vi "Write Arbs.vi"(8 "error in (no error)":errorcluster, 10 "Arbs":T1[](array[typedef]), 11 "ArbitraryFunction in":refnum<class "ArbitraryFunction.lvclass">) -> (0 "error out":errorcluster, 3 "ArbitraryFunction out":refnum<class "ArbitraryFunction.lvclass">)   [LabVIEW 2014, in "Functions.lvlib" / "ArbitraryFunction.lvclass"]
uses:
  ArbitraryFunction.lvclass
  TypeDefs/Arbitrary.ctl
  ArbitraryFunction.lvclass/ArbitraryFunction.ctl
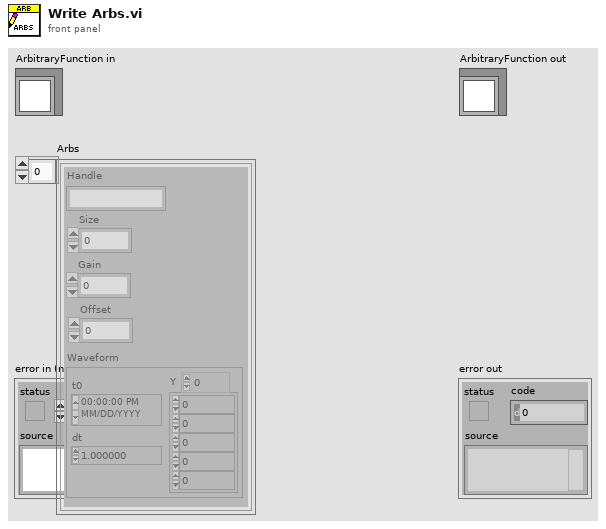
[diagram p1: front panel]
types:
  T1 = typedef "Functions.lvlib/ArbitraryFunction.lvclass/Arbitrary.ctl" = cluster{"Handle":string, "Size":i32, "Gain":dbl, "Offset":dbl, "Waveform":waveform(dbl)}
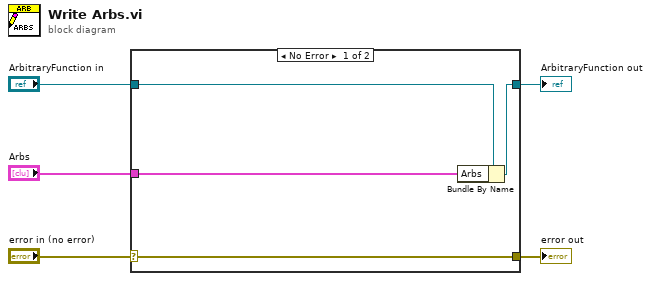
[diagram p0: block diagram]
diagram:
  n1 = case shown="No Error" "error in (no error)" {
    selector: "error in (no error)" -> [w9 w10]
    tunnel: [w9 w10] -> w4
    tunnel: [w7 w11] -> w2
    tunnel: "ArbitraryFunction in" -> [w8 w11]
    tunnel: "Arbs" -> [w6 _]
    frame No Error {
      n2 = Bundle By Name(cluster=w8, "Arbs"=w6) -> (w7:refnum<class "ArbitraryFunction.lvclass">)
    }
    frame Error {
    }
  }
  "error out" <- w4
  "ArbitraryFunction out" <- w2
